vi "Vision Research Phantom Series PhFile PhGetCineLive.vi"(0 "CN (in)":u32, 5 "Error In (no error)":errorcluster) -> (14 "CN (out)":u32, 15 "pCH (out)":u32, 19 "Error Out":errorcluster)   [LabVIEW 2013, in "VRI.lvlib"]
doc: "PhGetCineLive\nHRESULT PhGetCineLive(INT CN, PCINEHANDLE pCH);\n\nParameters\nCN [in]\n Camera number the requested live cine belongs to.\npCH [out]\n Pointer where to store live cine handle.\n\nReturn Value\nThe function returns ERR_Ok in case of success or an error code, otherwise. To get extended error information call PhGetErrorMessage.\n\nRemarks\nReturns the cinehandle corresponding to the live cine for the given camera. The live cine main use is reading live images from a certain camera. However, it can be used like any other cine as well; for example, for setting images processing parameters.\nPlease note that the live cinehandle is automatically created and automatically destructed. PhGetCineLive is used just for obtaining this already allocated and initialized cinehandle. \nPhDestroyCine must not be called for a live cine.\n\nRequired Header\nPhFile.h"
uses:
  VRI.lvlib
  Phantom DLLs/PhFile.Dll
panel:
  # "For instructions on the use of this VI, press Ctrl+H to display the help window and move the mouse over the icon, controls, and indicators"
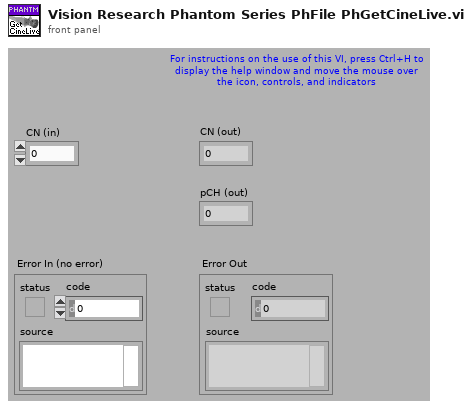
[diagram p1: front panel]
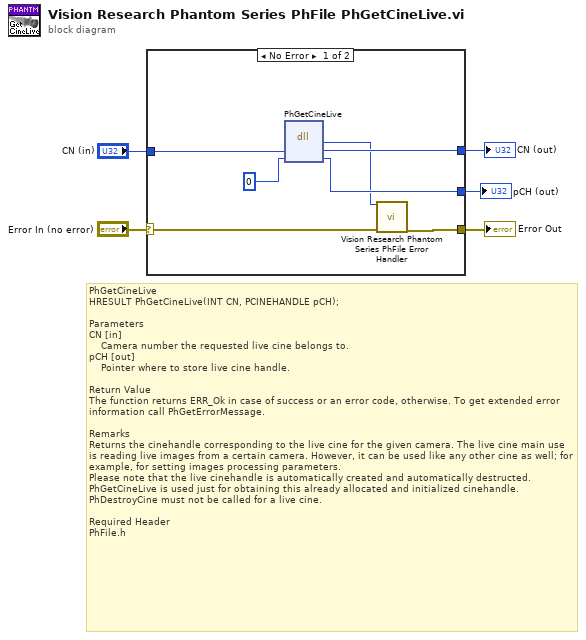
[diagram p0: block diagram]
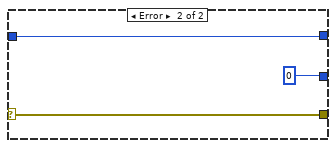
[diagram p2: hidden frame]
diagram:
  # "PhGetCineLive\nHRESULT PhGetCineLive(INT CN, PCINEHANDLE pCH);\n\nParameters\nCN [in]\n    Camera number the requested live cine belongs to.\npCH [out]\n    Pointer where to store live cine handle.\n\nReturn Value\nThe function returns ERR_Ok in case of success or an error code, otherwise. To get extended error information call PhGetErrorMessage.\n\nRemarks\nReturns the cinehandle corresponding to the live cine for the given camera. The live cine main use is reading live images from a certain camera. However, it can be used like any other cine as well; for example, for setting images processing parameters.\nPlease note that the live cinehandle is automatically created and automatically destructed. PhGetCineLive is used just for obtaining this already allocated and initialized cinehandle. \nPhDestroyCine must not be called for a live cine.\n\nRequired Header\nPhFile.h"
  n1 = case shown="No Error" "Error In (no error)" {
    selector: "Error In (no error)" -> [w12 w15]
    tunnel: [w11 w15] -> w4
    tunnel: "CN (in)" -> [w10 w14]
    tunnel: [w9 w14] -> w2
    tunnel: [w8 0] -> w1
    frame No Error {
      n2 = dll-call lib="C:/Projects/SDK/64-bit/Vision Research Phantom Series Labview Driver/Phantom DLLs/PhFile.dll" fn="PhGetCineLive"("CN"=w10, "pCH"=0) -> ("HRESULT"=w6:i32, "CN"=w9:i32, "pCH"=w8:u32)  [unwired: 3 in, 2 out]
      n3 = call "Vision Research Phantom Series PhFile Error Handler.vi"("Error Code (0)"=w6, "Error In (no error)"=w12) -> ("Error Out"=w11:errorcluster)  [unwired: 17 out]
    }
    frame Error {
    }
  }
  "Error Out" <- w4
  "CN (out)" <- w2
  "pCH (out)" <- w1
